vi "solar_voy_demo Test Packets.vi"() -> ()   [LabVIEW 2018]
doc: "This example exports native and custom packets."
panel:
  in  "TARGET":string
  in  "CMD":enum8{"CMD", "TLM"}(ring)
  in  "Tree":string(tree)
  in  "Select Packets":T1(ring)
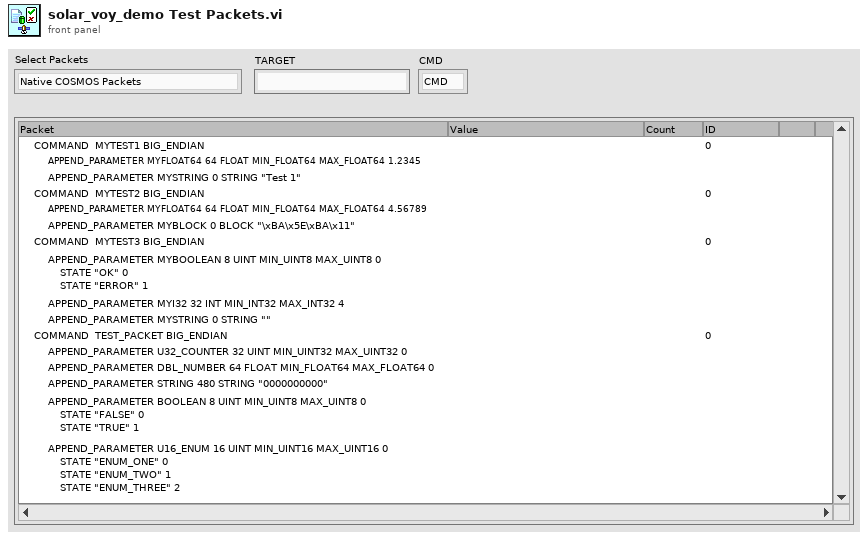
[diagram p1: front panel]
types:
  T1 = enum16{"Native COSMOS Packets", "Native COSMOS Array Packets", "Native COSMOS Array Packets Fixed", "Custom LabVIEW Packets", "Custom Test Packets"}
  T2 = cluster{"Native COSMOS Packets":cluster{"MYUINT8":cluster{"VALUE":u8}, "MYUINT16":cluster{"VALUE":u16}, "MYUINT32":cluster{"VALUE":u32}, "MYUINT64":cluster{"VALUE":u64}, "MYINT8":cluster{"VALUE":i8}, "MYINT16":cluster{"VALUE":i16}, "MYINT32":cluster{"VALUE":i32}, "MYINT64":cluster{"VALUE":i64}, "MYFLOAT32":cluster{"VALUE":sgl}, "MYFLOAT64":cluster{"VALUE":dbl}, "MYSTRING":cluster{"VALUE":string}, "MYBLOCK":cluster{"VALUE,t=block":string}}, "Native COSMOS Array Packets":cluster{"MYUINT8_1D":cluster{"VALUE":u8[]}, "MYUINT16_1D":cluster{"VALUE":u16[]}, "MYUINT32_1D":cluster{"VALUE":u32[]}, "MYUINT64_1D":cluster{"VALUE":u64[]}, "MYINT8_1D":cluster{"VALUE":i8[]}, "MYINT16_1D":cluster{"VALUE":i16[]}, "MYINT32_1D":cluster{"VALUE":i32[]}, "MYINT64_1D":cluster{"VALUE":i64[]}, "MYFLOAT32_1D":cluster{"VALUE":sgl[]}, "MYFLOAT64_1D":cluster{"VALUE":dbl[]}, "MYSTRING_1D":cluster{"VALUE":string[]}, "MYBLOCK_1D":cluster{"VALUE,t=block":string[]}}, "Native COSMOS Array Packets Fixed":cluster{"MYUINT8_1D":cluster{"VALUE,b=24":u8[]}, "MYUINT16_1D":cluster{"VALUE,b=48":u16[]}, "MYUINT32_1D":cluster{"VALUE,b=96":u32[]}, "MYUINT64_1D":cluster{"VALUE,b=192":u64[]}, "MYINT8_1D":cluster{"VALUE,b=24":i8[]}, "MYINT16_1D":cluster{"VALUE,b=48":i16[]}, "MYINT32_1D":cluster{"VALUE,b=96":i32[]}, "MYINT64_1D":cluster{"VALUE,b=192":i64[]}, "MYFLOAT32_1D":cluster{"VALUE,b=128":sgl[]}, "MYFLOAT64_1D":cluster{"VALUE,b=256":dbl[]}, "MYSTRING_1D":cluster{"VALUE,b=352,e=88":string[]}, "MYBLOCK_1D":cluster{"VALUE,t=block,b=192,e=48":string[]}}, "Custom LabVIEW Packets":cluster{"MYUINT8_ENUM":cluster{"VALUE":enum8{"ITEM1", "ITEM2", "ITEM3"}}, "MYUINT16_ENUM":cluster{"VALUE":enum16{"CAT", "DOG", "BIRD", "MOOSE"}}, "MYUINT32_ENUM":cluster{"VALUE":enum32{"ryan", "susan", "steve", "larry", "smith", "joe"}}, "MYBOOLEAN":cluster{"VALUE,s=OFF|ON":bool}, "MYSTRING_FIXED":cluster{"VALUE,b=24":string}, "MYBLOCK_FIXED":cluster{"VALUE,t=block,b=32":string}, "MYPATH":cluster{"VALUE":path}}, "Custom Test Packets":cluster{"MYTEST1":cluster{"MYFLOAT64":dbl, "MYSTRING":string}, "MYTEST2":cluster{"MYFLOAT64":dbl, "MYBLOCK,t=block":string}, "MYTEST3":cluster{"MYBOOLEAN,s=OK|ERROR":bool, "MYI32":i32, "MYSTRING":string}, "TEST_PACKET":cluster{"U32_COUNTER":u32, "DBL_NUMBER":dbl, "STRING,b=480":string, "BOOLEAN":bool, "U16_ENUM":enum16{"ENUM_ONE", "ENUM_TWO", "ENUM_THREE"}, "U8_RING":u8, "U32_ARRAY,e=5":u32[], "U8":u32}}}
  T3 = cluster{"MYUINT8":cluster{"VALUE":u8}, "MYUINT16":cluster{"VALUE":u16}, "MYUINT32":cluster{"VALUE":u32}, "MYUINT64":cluster{"VALUE":u64}, "MYINT8":cluster{"VALUE":i8}, "MYINT16":cluster{"VALUE":i16}, "MYINT32":cluster{"VALUE":i32}, "MYINT64":cluster{"VALUE":i64}, "MYFLOAT32":cluster{"VALUE":sgl}, "MYFLOAT64":cluster{"VALUE":dbl}, "MYSTRING":cluster{"VALUE":string}, "MYBLOCK":cluster{"VALUE,t=block":string}}
  T4 = cluster{"MYUINT8_1D":cluster{"VALUE":u8[]}, "MYUINT16_1D":cluster{"VALUE":u16[]}, "MYUINT32_1D":cluster{"VALUE":u32[]}, "MYUINT64_1D":cluster{"VALUE":u64[]}, "MYINT8_1D":cluster{"VALUE":i8[]}, "MYINT16_1D":cluster{"VALUE":i16[]}, "MYINT32_1D":cluster{"VALUE":i32[]}, "MYINT64_1D":cluster{"VALUE":i64[]}, "MYFLOAT32_1D":cluster{"VALUE":sgl[]}, "MYFLOAT64_1D":cluster{"VALUE":dbl[]}, "MYSTRING_1D":cluster{"VALUE":string[]}, "MYBLOCK_1D":cluster{"VALUE,t=block":string[]}}
  T5 = cluster{"MYUINT8_1D":cluster{"VALUE,b=24":u8[]}, "MYUINT16_1D":cluster{"VALUE,b=48":u16[]}, "MYUINT32_1D":cluster{"VALUE,b=96":u32[]}, "MYUINT64_1D":cluster{"VALUE,b=192":u64[]}, "MYINT8_1D":cluster{"VALUE,b=24":i8[]}, "MYINT16_1D":cluster{"VALUE,b=48":i16[]}, "MYINT32_1D":cluster{"VALUE,b=96":i32[]}, "MYINT64_1D":cluster{"VALUE,b=192":i64[]}, "MYFLOAT32_1D":cluster{"VALUE,b=128":sgl[]}, "MYFLOAT64_1D":cluster{"VALUE,b=256":dbl[]}, "MYSTRING_1D":cluster{"VALUE,b=352,e=88":string[]}, "MYBLOCK_1D":cluster{"VALUE,t=block,b=192,e=48":string[]}}
  T6 = cluster{"MYUINT8_ENUM":cluster{"VALUE":enum8{"ITEM1", "ITEM2", "ITEM3"}}, "MYUINT16_ENUM":cluster{"VALUE":enum16{"CAT", "DOG", "BIRD", "MOOSE"}}, "MYUINT32_ENUM":cluster{"VALUE":enum32{"ryan", "susan", "steve", "larry", "smith", "joe"}}, "MYBOOLEAN":cluster{"VALUE,s=OFF|ON":bool}, "MYSTRING_FIXED":cluster{"VALUE,b=24":string}, "MYBLOCK_FIXED":cluster{"VALUE,t=block,b=32":string}, "MYPATH":cluster{"VALUE":path}}
  T7 = cluster{"MYTEST1":cluster{"MYFLOAT64":dbl, "MYSTRING":string}, "MYTEST2":cluster{"MYFLOAT64":dbl, "MYBLOCK,t=block":string}, "MYTEST3":cluster{"MYBOOLEAN,s=OK|ERROR":bool, "MYI32":i32, "MYSTRING":string}, "TEST_PACKET":cluster{"U32_COUNTER":u32, "DBL_NUMBER":dbl, "STRING,b=480":string, "BOOLEAN":bool, "U16_ENUM":enum16{"ENUM_ONE", "ENUM_TWO", "ENUM_THREE"}, "U8_RING":u8, "U32_ARRAY,e=5":u32[], "U8":u32}}
  T8 = typedef "solar_voy_def_ctl PACKET.ctl" = cluster{"PACKET_ID":T9, "ENDIAN":enum8{"BIG", "LITTLE"}, "DESC":string, "HZRD":bool, "ITEMS":T10[], "NoExport":bool, "last_time":timestamp, "last_count":u32, "last_data":string}
  T9 = typedef "solar_voy_def_ctl PACKET_ID.ctl" = cluster{"ID":u16, "CMD":enum8{"CMD", "TLM"}, "TARGET":string, "PACKET":string}
  T10 = typedef "solar_voy_def_ctl ITEM.ctl" = cluster{"NAME":string, "OFFSET":i32, "SIZE":i32, "TYPE":T11, "EACH_SIZE":i32, "LVTYPE":T12, "MIN":dbl, "MAX":dbl, "DEFAULT":string, "DESC":string, "ID":bool, "MODIFIERS":variant, "last_value":variant}
  T11 = typedef "solar_voy_def_ctl ITEM TYPE.ctl" = enum8{"BLOCK", "INT", "UINT", "FLOAT", "STRING"}
  T12 = typedef "solar_type Item Type.ctl" = enum16{"NULL", "UNKNOWN", "CLUSTER", "I8", "I16", "I32", "I64", "U8", "U16", "U32", "U64", "U8_ENUM", "U16_ENUM", "U32_ENUM", "SGL", "DBL", "BOOLEAN", "STRING", "PATH", "VISA", "TAG", "TIME", "I8_1D", "I16_1D", "I32_1D", "I64_1D", "U8_1D", "U16_1D", "U32_1D", "U64_1D", "U8_ENUM_1D", "U16_ENUM_1D", "U32_ENUM_1D", "SGL_1D", "DBL_1D", "BOOLEAN_1D", "STRING_1D", "PATH_1D", "VISA_1D", "TAG_1D", "TIME_1D", "I8_2D", "I16_2D", "I32_2D", "I64_2D", "U8_2D", "U16_2D", "U32_2D", "U64_2D", "U8_ENUM_2D", "U16_ENUM_2D", "U32_ENUM_2D", "SGL_2D", "DBL_2D", "BOOLEAN_2D", "STRING_2D", "PATH_2D", "VISA_2D", "TAG_2D", "TIME_2D"}
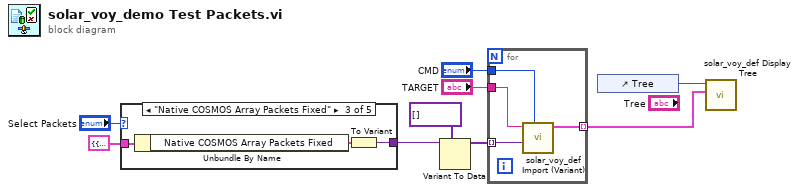
[diagram p0: block diagram]
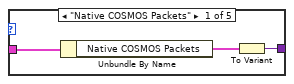
[diagram p2: hidden frame]
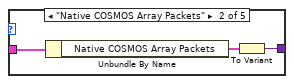
[diagram p3: hidden frame]
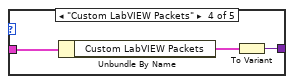
[diagram p4: hidden frame]
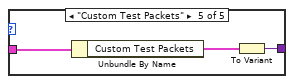
[diagram p5: hidden frame]
diagram:
  n1 = case shown="\"Native COSMOS Array Packets Fixed\"" "Select Packets" {
    tunnel: T2 {"Native COSMOS Packets"={"MYUINT8"={"VALUE"=255}, "MYUINT16"={"VALUE"=65535}, "MYUINT32"={"VALUE"=4294967295}, "MYUINT64"={"VALUE"=18446744073709551615}, "MYINT8"={"VALUE"=-128}, "MYINT16"={"VALUE"=-32768}, "MYINT32"={"VALUE"=-2147483648}, "MYINT64"={"VALUE"=-9223372036854775808}, "MYFLOAT32"={"VALUE"=3.141563}, "MYFLOAT64"={"VALUE"=-1.234567891e-05}, "MYSTRING"={"VALUE"="Hello World"}, "MYBLOCK"={"VALUE,t=block"="Þ­¾ï"}}, "Native COSMOS Array Packets"={"MYUINT8_1D"={"VALUE"=[255, 0, 5]}, "MYUINT16_1D"={"VALUE"=[65535, 0, 50]}, "MYUINT32_1D"={"VALUE"=[4294967295, 0, 500]}, "MYUINT64_1D"={"VALUE"=[18446744073709551615, 0, 5000]}, "MYINT8_1D"={"VALUE"=[127, -128, -5]}, "MYINT16_1D"={"VALUE"=[32767, -32768, -50]}, "MYINT32_1D"={"VALUE"=[2147483647, -2147483648, -500]}, "MYINT64_1D"={"VALUE"=[9223372036854775807, -9223372036854775808, -5000]}, "MYFLOAT32_1D"={"VALUE"=[-1.234567, inf, -inf, nan]}, "MYFLOAT64_1D"={"VALUE"=[123456789.12345679, inf, -inf, nan]}, "MYSTRING_1D"={"VALUE"=["Please, set", "Me Free", "Good", "Bad\u0000ignore"]}, "MYBLOCK_1D"={"VALUE,t=block"=["\u0000\u0001\u0002", "Eg‰«Íï", "ÿÿÿÿ", "\u0000\u0000\u0000\u0000\u0000"]}}, "Native COSMOS Array Packets Fixed"={"MYUINT8_1D"={"VALUE,b=24"=[255, 0, 5]}, "MYUINT16_1D"={"VALUE,b=48"=[65535, 0, 50]}, "MYUINT32_1D"={"VALUE,b=96"=[4294967295, 0, 500]}, "MYUINT64_1D"={"VALUE,b=192"=[18446744073709551615, 0, 5000]}, "MYINT8_1D"={"VALUE,b=24"=[127, -128, -5]}, "MYINT16_1D"={"VALUE,b=48"=[32767, -32768, -50]}, "MYINT32_1D"={"VALUE,b=96"=[2147483647, -2147483648, -500]}, "MYINT64_1D"={"VALUE,b=192"=[9223372036854775807, -9223372036854775808, -5000]}, "MYFLOAT32_1D"={"VALUE,b=128"=[-1.234567, inf, -inf, nan]}, "MYFLOAT64_1D"={"VALUE,b=256"=[123456789.12345679, inf, -inf, nan]}, "MYSTRING_1D"={"VALUE,b=352,e=88"=["Please, set", "Me Free", "Good", "Bad\u0000ignore"]}, "MYBLOCK_1D"={"VALUE,t=block,b=192,e=48"=["\u0000\u0001\u0002", "Eg‰«Íï", "ÿÿÿÿ", "\u0000\u0000\u0000\u0000\u0000"]}}, "Custom LabVIEW Packets"={"MYUINT8_ENUM"={"VALUE"=enum."ITEM2"}, "MYUINT16_ENUM"={"VALUE"=enum."BIRD"}, "MYUINT32_ENUM"={"VALUE"=enum."joe"}, "MYBOOLEAN"={"VALUE,s=OFF|ON"=FALSE}, "MYSTRING_FIXED"={"VALUE,b=24"="CAR"}, "MYBLOCK_FIXED"={"VALUE,t=block,b=32"="\u0001\u0002\u0003\u0004"}, "MYPATH"={"VALUE"=path "C:/Data/test.txt"}}, "Custom Test Packets"={"MYTEST1"={"MYFLOAT64"=1.2345, "MYSTRING"="Test 1"}, "MYTEST2"={"MYFLOAT64"=4.56789, "MYBLOCK,t=block"="º^º\u0011"}, "MYTEST3"={"MYBOOLEAN,s=OK|ERROR"=FALSE, "MYI32"=4, "MYSTRING"=""}, "TEST_PACKET"={"U32_COUNTER"=0, "DBL_NUMBER"=0.0, "STRING,b=480"="0000000000", "BOOLEAN"=FALSE, "U16_ENUM"=enum."ENUM_ONE", "U8_RING"=0, "U32_ARRAY,e=5"=[], "U8"=0}}} ("Test Packets") -> [w12 w15 w18 w21 w24]
    tunnel: [w10 w13 w16 w19 w22] -> w7
    frame "Native COSMOS Packets" {
      n2 = Unbundle By Name(w12) -> ("Native COSMOS Packets"=w11:T3)
      n3 = To Variant(anything=w11) -> (Variant=w10:variant)
    }
    frame "Native COSMOS Array Packets" {
      n4 = Unbundle By Name(w15) -> ("Native COSMOS Array Packets"=w14:T4)
      n5 = To Variant(anything=w14) -> (Variant=w13:variant)
    }
    frame "Native COSMOS Array Packets Fixed" {
      n6 = Unbundle By Name(w18) -> ("Native COSMOS Array Packets Fixed"=w17:T5)
      n7 = To Variant(anything=w17) -> (Variant=w16:variant)
    }
    frame "Custom LabVIEW Packets" {
      n8 = Unbundle By Name(w21) -> ("Custom LabVIEW Packets"=w20:T6)
      n9 = To Variant(anything=w20) -> (Variant=w19:variant)
    }
    frame "Custom Test Packets" {
      n10 = Unbundle By Name(w24) -> ("Custom Test Packets"=w23:T7)
      n11 = To Variant(anything=w23) -> (Variant=w22:variant)
    }
  }
  n12 = Variant To Data(type=variant[] [], Variant=w7) -> (data=w8:variant[])  [unwired: 1 in, 1 out]
  n13 = for {
    tunnel: w8 -> [w26] mode=indexing
    tunnel: [w28] -> w4 mode=indexing
    tunnel: "TARGET" -> [w27]
    tunnel: "CMD" -> [w25]
    n14 = call "solar_voy_def Import (Variant).vi"("CMD"=w25, "Variant"=w26, "TARGET"=w27) -> ("PACKET"=w28:T8)  [unwired: 7 in, 1 out]
  }
  n15 = control-ref of="Tree"() -> (w5:refnum<vi>)
  n16 = call "solar_voy_def Display Tree.vi"("PACKETS"=w4, "Tree Refnum"=w5) -> ()  [unwired: 9 in, 1 out]
